vi "getTrigger.vi"(8 "error in (no error)":errorcluster, 11 "Refnum in":refnum<k21>) -> (0 "error out":errorcluster, 2 "triggered":bool, 3 "Refnum out":refnum<k21>)   [LabVIEW 2011]
uses:
  C:/Program Files/National Instruments/LabVIEW 2011/resource/objmgr/daqmx.rc
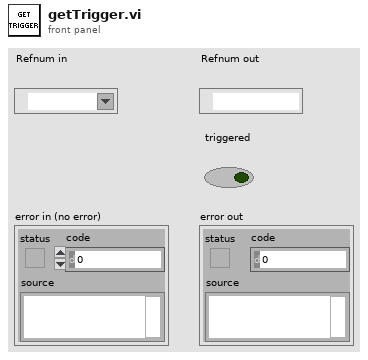
[diagram p1: front panel]
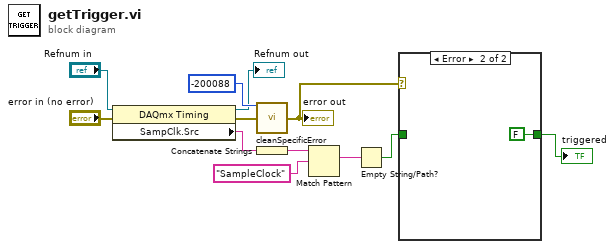
[diagram p0: block diagram]
diagram:
  n1 = property class="DAQmx Timing"(reference="Refnum in", error in="error in (no error)") -> (reference out=→"Refnum out":refnum<k21>, error out=w10:errorcluster, "SampClk.Src"=w7:tag)
  n2 = call "cleanSpecificError.vi"("error out"=w10, "error code"=-200088) -> ("error IO"=w3:errorcluster)  [unwired: 2 in, 1 out]
  "error out" <- w3
  n3 = Concatenate Strings(w7) -> (w6:string)
  n4 = Match Pattern(string=w6, regular expression="SampleClock") -> (match substring=w4:string)  [unwired: 1 in, 3 out]
  n5 = Empty String/Path?(string/path=w4) -> (empty?=w2:bool)
  n6 = case shown="Error" w3 {
    tunnel: w2 -> [w13 _]
    tunnel: [w13 FALSE] -> w1
    frame No Error {
    }
    frame Error {
    }
  }
  "triggered" <- w1
